vi "convertObjectToCluster.vi"(0 "Object in":refnum<class>, 1 "error in":errorcluster) -> (14 "VCluster":variant, 15 "error out":errorcluster)   [LabVIEW 2020, in "JKI JSON Object Serialization.lvlib" / "OOP_Utility.lvlib"]
doc: "Transform object to a flat cluster containing all elements from every class in the hierarchy.\n\nGCraftsman JSON Object Serialization Toolkit\nwww.GCraftsman.com\nCopyright (c) 2017, GCraftsman"
uses:
  OOP_Utility.lvlib
  Reflection/Assert No Duplicate Named Private Data Elements.vi/91249ab7-5ea3-4d6c-b8df-29db4c9f394f.vi
  Reflection/Assert No Duplicate Named Private Data Elements.vi/f7c1a62c-1232-4a35-ba9e-0fa75d385864.vi
  <vilib>/AdvancedString/1D String Array to Delimited String.vi
  <vilib>/dlg_ctls.llb/Space Constant.vi
  Reflection/Assert No Duplicate Named Private Data Elements.vi/91249ab7-5ea3-4d6c-b8df-29db4c9f394f.vi/73eff78f-802f-4e82-99e6-5ec6d44c8b1c.vi
  Reflection/Assert No Duplicate Named Private Data Elements.vi/91249ab7-5ea3-4d6c-b8df-29db4c9f394f.vi/a79ef678-9021-4176-8e9d-ef71acec083e.vi
  Reflection/Assert No Duplicate Named Private Data Elements.vi/91249ab7-5ea3-4d6c-b8df-29db4c9f394f.vi/6194b64b-8f19-4369-9ca4-18e99c56e175.vi
  Reflection/Assert No Duplicate Named Private Data Elements.vi/91249ab7-5ea3-4d6c-b8df-29db4c9f394f.vi/4000f349-3ba7-45cd-93a4-b1a8967d5605.vi
  Reflection/reflectionPool.vi
  <userlib>/_OpenG.lib/lvdata/lvdata.llb/Get Cluster Element Names__ogtk.vi
  <vilib>/Utility/error.llb/Error Cluster From Error Code.vi
  Reflection/Reflection.lvclass
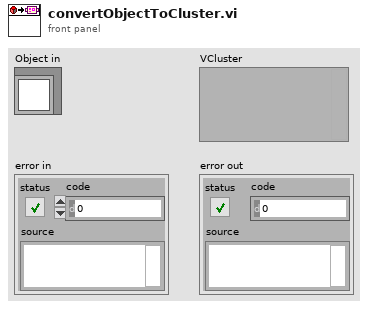
[diagram p1: front panel]
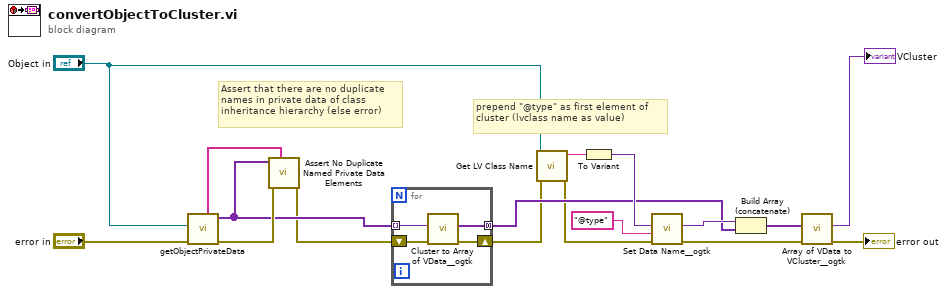
[diagram p0: block diagram]
diagram:
  # "prepend \"@type\" as first element of cluster (lvclass name as value)"
  # "Assert that there are no duplicate names in private data of class inheritance hierarchy (else error)"
  n1 = call "getObjectPrivateData.vi"("error in (no error)"="error in", "object in"="Object in") -> ("error out"=w16:errorcluster, "private data"=w7:variant[], "interitance classes"=w4:string[])  [unwired: 6 in, 1 out]
  n2 = call "Assert No Duplicate Named Private Data Elements.vi"("class names"=w4, "error in"=w16, "private data clusters"=w7) -> ("error out"=w5:errorcluster)  [unwired: 8 in]
  n3 = for {
    tunnel: w7 -> [w19] mode=indexing
    tunnel: [w20] -> w6 mode=concatenating
    shift-right: [w21] -> w2
    shift-left: w5 -> [w18]
    n4 = call <userlib>:"Cluster to Array of VData__ogtk.vi"("error in (no error)"=w18, "Cluster"=w19) -> ("error out"=w21:errorcluster, "Array of VData"=w20:variant[])  [unwired: 8 in]
  }
  n5 = call <vilib>:"Get LV Class Name.vi"("error in (no error)"=w2, "object"="Object in") -> ("error out"=w1:errorcluster, "class name"=w13:string)  [unwired: 8 in]
  n6 = To Variant(anything=w13) -> (Variant=w12:variant)
  n7 = call <userlib>:"Set Data Name__ogtk.vi"("error in (no error)"=w1, "Data Name"="@type", "Data"=w12) -> ("error out"=w8:errorcluster, "Renamed Data"=w10:variant)  [unwired: 7 in]
  n8 = Build Array (concatenate)(w10, w6) -> (w9:variant[])
  n9 = call <userlib>:"Array of VData to VCluster__ogtk.vi"("error in (no error)"=w8, "Array"=w9) -> ("error out"=→"error out":errorcluster, "VCluster"=→"VCluster":variant)  [unwired: 8 in]
